vi "SET_Origin.vi"(8 "error in (no error)":errorcluster, 10 "Point32":T1, 11 "Layer.lvclass in":refnum<class "Layer.lvclass">) -> (0 "error out":errorcluster, 3 "Layer.lvclass out":refnum<class "Layer.lvclass">)   [LabVIEW 2021, in "Layer.lvclass"]
doc: "Specify the Origin of the User Layer."
uses:
  <vilib>/LabVIEW Icon API/lv_icon/Classes/Layer/Layer.lvclass
  <vilib>/Utility/miscctls.llb/LVPoint32TypeDef.ctl
  <vilib>/LabVIEW Icon API/lv_icon/Classes/Layer/Layer.lvclass/Layer.ctl
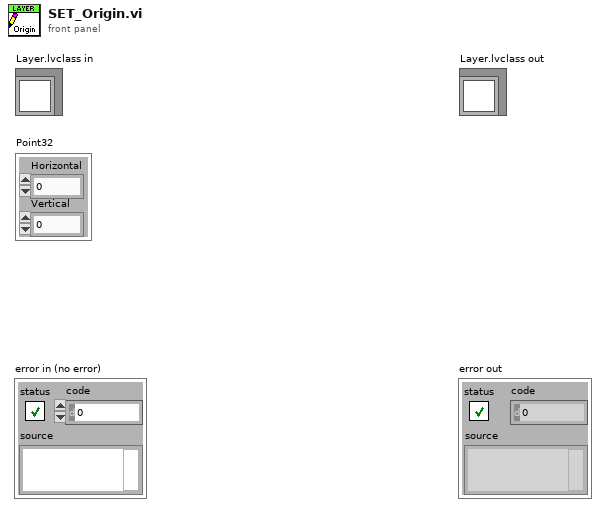
[diagram p1: front panel]
types:
  T1 = typedef "LVPoint32TypeDef.ctl" = cluster{"Horizontal":i32, "Vertical":i32}
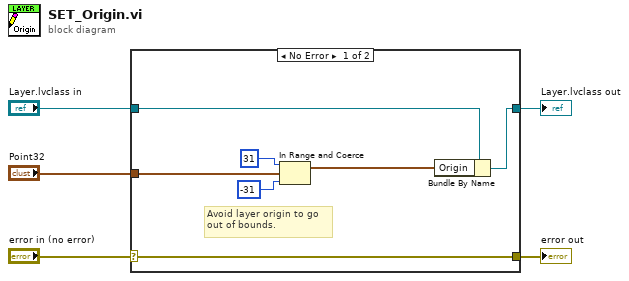
[diagram p0: block diagram]
diagram:
  n1 = case shown="No Error" "error in (no error)" {
    selector: "error in (no error)" -> [w12 w13]
    tunnel: [w12 w13] -> w4
    tunnel: [w10 w14] -> w2
    tunnel: "Layer.lvclass in" -> [w11 w14]
    tunnel: "Point32" -> [w7 _]
    frame No Error {
      # "Avoid layer origin to go\nout of bounds."
      n2 = In Range and Coerce(upper limit=31, x=w7, lower limit=-31) -> (coerced(x)=w6:T1)  [unwired: 1 out]
      n3 = Bundle By Name(cluster=w11, "Origin"=w6) -> (w10:refnum<class "Layer.lvclass">)
    }
    frame Error {
    }
  }
  "error out" <- w4
  "Layer.lvclass out" <- w2
